vi "Add Stack Frame.vi"(8 "error in (no error)":errorcluster, 9 "Return Bindings":string[](array[string]), 10 "New PC":i32=-1, 11 "gScript Interpreter in":refnum<class "gScript Interpreter.lvclass">) -> (0 "error out":errorcluster, 3 "gScript Interpreter out":refnum<class "gScript Interpreter.lvclass">)   [LabVIEW 2017, in "gScript Interpreter.lvclass"]
uses:
  gScript Interpreter.lvclass
  gScript Interpreter.lvclass/gScript Interpreter.ctl
  Type Definitions/Stack Frame.ctl
  Type Definitions/Variable Table.ctl
  Type Definitions/Variable.ctl
  Type Definitions/Memory Cell.ctl
  Type Definitions/Memory Cell Type Enum.ctl
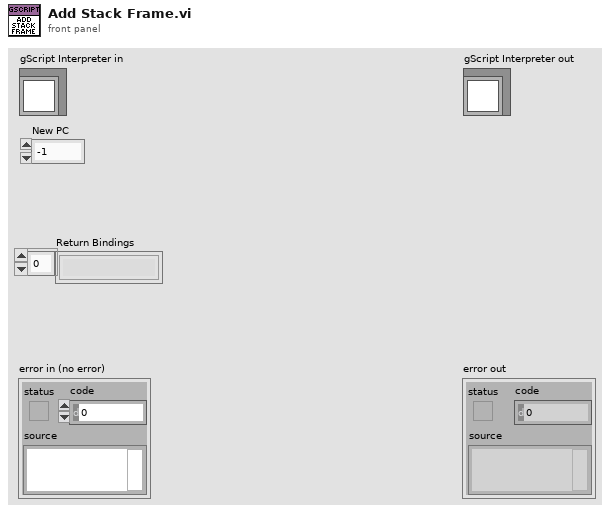
[diagram p1: front panel]
types:
  T1 = typedef "Stack Frame.ctl" = cluster{"Variable Table":T2, "Return Pointer":i32, "Return Bindings":string[]}
  T2 = typedef "Variable Table.ctl" = T3[]
  T3 = typedef "Variable.ctl" = cluster{"Variable Name":string, "Memory Cell":T4}
  T4 = typedef "Memory Cell.ctl" = cluster{"type":T5, "x":dbl, "y":dbl, "z":dbl, "w":dbl}
  T5 = typedef "Memory Cell Type Enum.ctl" = enum16{"integer", "float", "vector", "rotation"}
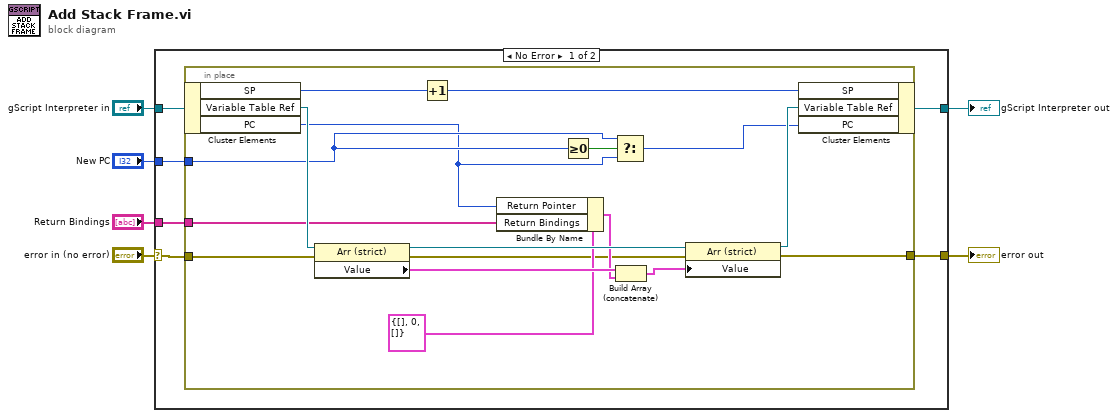
[diagram p0: block diagram]
diagram:
  n1 = case shown="No Error" "error in (no error)" {
    selector: "error in (no error)" -> [w11 w31]
    tunnel: [w9 w31] -> w5
    tunnel: [w10 w30] -> w3
    tunnel: "gScript Interpreter in" -> [w12 w30]
    tunnel: "New PC" -> [w8 _]
    tunnel: "Return Bindings" -> [w7 _]
    frame No Error {
      n2 = in-place {
        in-place-border: w11 -> [w28]
        in-place-border: [w18] -> w9
        in-place-border: w8 -> [w16]
        in-place-border: w7 -> [w14]
        n3 = in-place-cluster #1(w12) -> ("SP"=w27:i32, "Variable Table Ref"=w29:refnum<vi>, "PC"=w13:i32)
        n4 = property class="Arr (strict)"(reference=w29, error in=w28) -> (reference out=w23:refnum<vi>, error out=w19:errorcluster, "Value"=w25:T1[])
        n5 = Increment(x=w27) -> (x+1=w26:i32)
        n6 = Bundle By Name(cluster=T1 {"Variable Table"=[], "Return Pointer"=0, "Return Bindings"=[]} ("Stack Frame"), "Return Pointer"=w13, "Return Bindings"=w14) -> (w20:T1)
        n7 = Greater Or Equal To 0?(x=w16) -> (x >= 0?=w17:bool)
        n8 = Select(t=w16, s=w17, f=w13) -> (s? t:f=w15:i32)
        n9 = Build Array (concatenate)(w25, w20) -> (w24:T1[])
        n10 = property class="Arr (strict)"(reference=w23, error in=w19, "Value"=w24) -> (reference out=w22:refnum<vi>, error out=w18:errorcluster)
        n11 = in-place-cluster #1("SP"=w26, "Variable Table Ref"=w22, "PC"=w15) -> (w10:refnum<class "gScript Interpreter.lvclass">)
      }
    }
    frame Error {
    }
  }
  "error out" <- w5
  "gScript Interpreter out" <- w3
